vi "Add Channel to All Plugins.vi"(7 "GUID (Default Channel)":string="03D3BB99-1485-13A6-561D1F898F032919", 8 "error in (no error)":errorcluster, 9 "Channel":T1, 10 "Channel Name":string, 11 "Item Ref in":T3 format="%.0x") -> (0 "error out":errorcluster, 3 "Item Ref out":T3 format="%.0x")   [LabVIEW 2017, in "DSF System Explorer.lvlib"]
uses:
  DSF System Explorer.lvlib
  <vilib>/NI Veristand/Custom Device API/Custom Device Item Ref.ctl
  <vilib>/NI Veristand/Custom Device API/Custom Device Channel.ctl
  <vilib>/NI Veristand/Custom Device API/Custom Device Channel Type.ctl
  <vilib>/NI Veristand/Custom Device API/Custom Device API.lvlib
  Shared/DSF Shared.lvlib
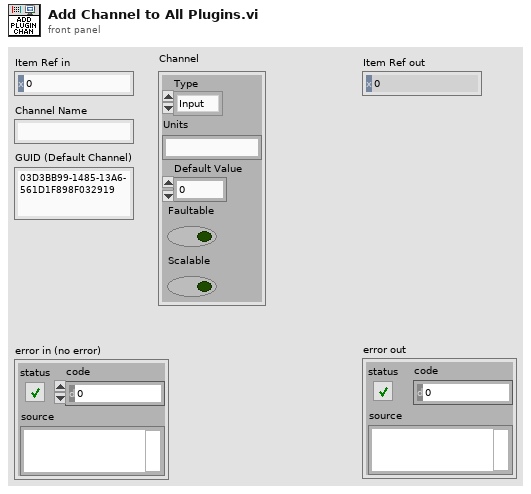
[diagram p1: front panel]
types:
  T1 = typedef "Custom Device API.lvlib/Custom Device Channel.ctl" = cluster{"Type":T2, "Units":string, "Default Value":dbl, "Faultable":bool, "Scalable":bool}
  T2 = typedef "Custom Device API.lvlib/Custom Device Channel Type.ctl" = enum16{"Input", "Output"}
  T3 = typedef "Custom Device API.lvlib/Custom Device Item Ref.ctl" = u64
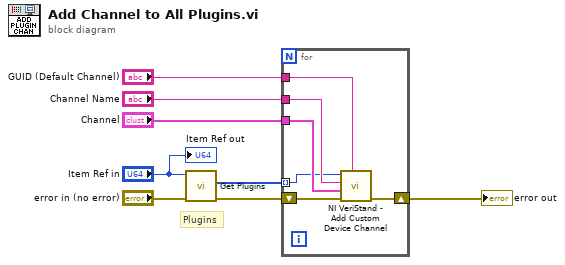
[diagram p0: block diagram]
diagram:
  # "Plugins"
  n1 = call "Get Plugins.vi"("error in (no error)"="error in (no error)", "Framework Ref in"="Item Ref in") -> ("error out"=w6:errorcluster, "Plugin refs"=w5:T3[])  [unwired: 7 in, 1 out]
  n2 = for {
    shift-right: [w13] -> w4
    shift-left: w6 -> [w14]
    tunnel: w5 -> [w10] mode=indexing
    tunnel: "Channel Name" -> [w11]
    tunnel: "Channel" -> [w12]
    tunnel: "GUID (Default Channel)" -> [w9]
    n3 = call <vilib>:"NI VeriStand - Add Custom Device Channel.vi"("GUID (Default Channel)"=w9, "error in (no error)"=w14, "Channel"=w12, "Channel Name"=w11, "Parent Ref in"=w10) -> ("error out"=w13:errorcluster)  [unwired: 3 in, 3 out]
  }
  "error out" <- w4
  "Item Ref out" <- "Item Ref in"
